vi "SetRegisterInitValue.vi"(0 "Index":i32, 1 "JSON":string="{}", 2 "Variant":variant, 5 "error in (no error)":errorcluster) -> (14 "<JSON>":string, 15 "Replaced":bool, 16 "Variant output":variant, 19 "error out":errorcluster)   [LabVIEW 2018]
uses:
  32b7ab6d-2b39-4956-83b2-5eda9bb9db11.vi
  <vilib>/JDP Science/JSONtext/Variant to JSON Text.vi
  <vilib>/JDP Science/JSONtext/JSONtext.lvlib
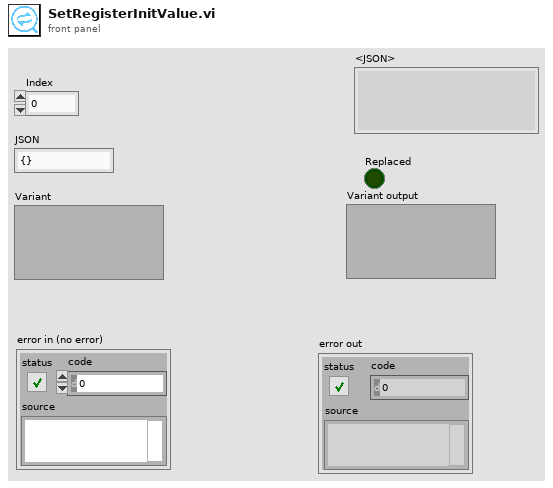
[diagram p1: front panel]
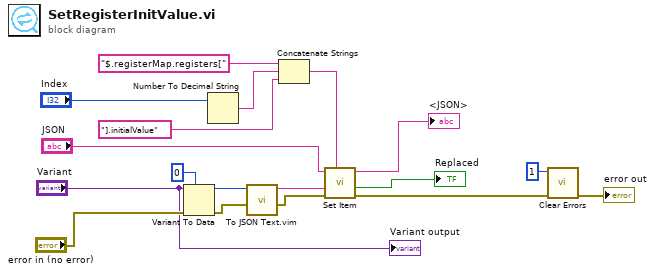
[diagram p0: block diagram]
diagram:
  n1 = Variant To Data(error in="error in (no error)", type=u64 0, Variant="Variant") -> (data=w12:u64, error out=w9:errorcluster)
  n2 = Number To Decimal String(number="Index") -> (decimal integer string=w15:string)  [unwired: 1 in]
  n3 = call "To JSON Text.vim"("error in (no error)"=w9, "Anything"=w12) -> ("error out"=w8:errorcluster, "<JSON>"=w13:string)  [unwired: 8 in]
  n4 = Concatenate Strings("$.registerMap.registers[" ("format string"), w15, "].initialValue") -> (w17:string)
  n5 = call <vilib>:"Set Item.vi"("$Path or Item Name"=w17, "error in (no error)"=w8, "JSON to Insert"=w13, "JSON"="JSON") -> ("error out"=w5:errorcluster, "Replaced"=→"Replaced":bool, "<JSON>"=→"<JSON>":string)  [unwired: 4 in]
  n6 = call <vilib>:"Clear Errors.vi"("error in (no error)"=w5, "specific error code to clear (0: all)"=1) -> ("error out"=→"error out":errorcluster)  [unwired: 4 in, 1 out]
  "Variant output" <- "Variant"
